vi "Log.vi"(8 "error in (no error)":errorcluster, 10 "tdms file":refnum<k34>, 11 "Acquired Result in":refnum<class "Acquired Result.lvclass">) -> (0 "error out":errorcluster, 2 "tdms file out":refnum<k34>, 3 "Acquired Result out":refnum<class "Acquired Result.lvclass">)   [LabVIEW 2016, in "Acquired Result.lvclass"]
uses:
  Acquired Result.lvclass
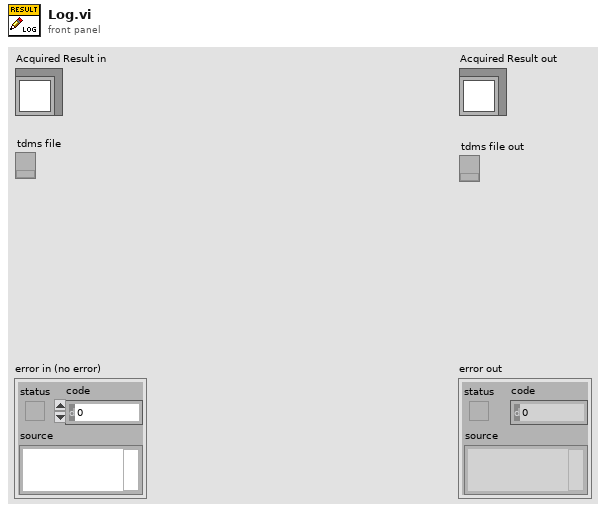
[diagram p1: front panel]
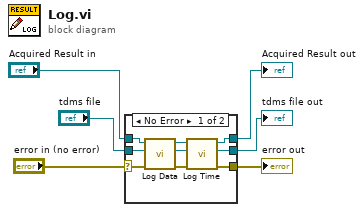
[diagram p0: block diagram]
diagram:
  n1 = case shown="No Error" "error in (no error)" {
    selector: "error in (no error)" -> [w11 w16]
    tunnel: "Acquired Result in" -> [w8 w18]
    tunnel: "tdms file" -> [w14 w17]
    tunnel: [w12 w17] -> w4
    tunnel: [w7 w18] -> w3
    tunnel: [w10 w16] -> w2
    frame No Error {
      n2 = call-dynamic "Log Data.vi"("error in (no error)"=w11, "tdms file"=w14, "Acquired Result in"=w8) -> ("error out"=w15:errorcluster, "tdms file out"=w13:refnum<k34>, "Acquired Result out"=w9:refnum<class "Acquired Result.lvclass">)  [unwired: 6 in]
      n3 = call-dynamic "Log Time.vi"("error in (no error)"=w15, "tdms file"=w13, "Acquired Result in"=w9) -> ("error out"=w10:errorcluster, "tdms file out"=w12:refnum<k34>, "Acquired Result out"=w7:refnum<class "Acquired Result.lvclass">)  [unwired: 6 in]
    }
    frame Error {
    }
  }
  "error out" <- w2
  "Acquired Result out" <- w3
  "tdms file out" <- w4
